vi "set_Ga_dilut.vi"(0 "Ga flow (0-10 sccm)":dbl, 1 "fDilution":dbl, 2 "Run":bool, 3 "Bubbler In":bool, 4 "Active":bool) -> ()   [LabVIEW 2011]
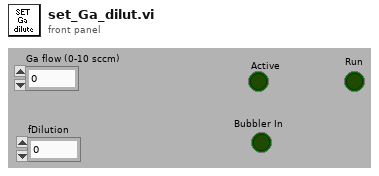
[diagram p1: front panel]
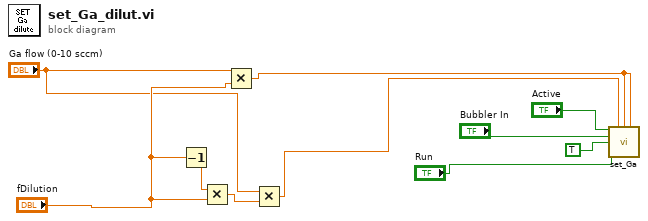
[diagram p0: block diagram]
diagram:
  n1 = Decrement(x="fDilution") -> (x-1=w6:dbl)
  n2 = Multiply(x=w6, y="fDilution") -> (x*y=w4:dbl)
  n3 = Multiply(x="Ga flow (0-10 sccm)", y="fDilution") -> (x*y=w1:dbl)
  n4 = Multiply(x="Ga flow (0-10 sccm)", y=w4) -> (x*y=w2:dbl)
  n5 = call "set_Ga.vi"("Ga Active"="Active", "Ga Flow 3"=w2, "Ga Flow 2"=w1, "Ga Flow 1"=w1, "Ga Bubbler"="Bubbler In", "Ga H2 Dilute"=TRUE, "Ga Run"="Run") -> ()  [unwired: 9 in]
